vi "parse and execute command.vi"(8 "Python Command":string) -> (1 "Python Return String":string, 2 "exit":bool)   [LabVIEW 2014]
panel:
  in  "base path":path=path "D:/Scripts/VIs/SLLServer/NanonisCommand"
  out "error out":errorcluster
  in  "VI Refnum":refnum<vi>
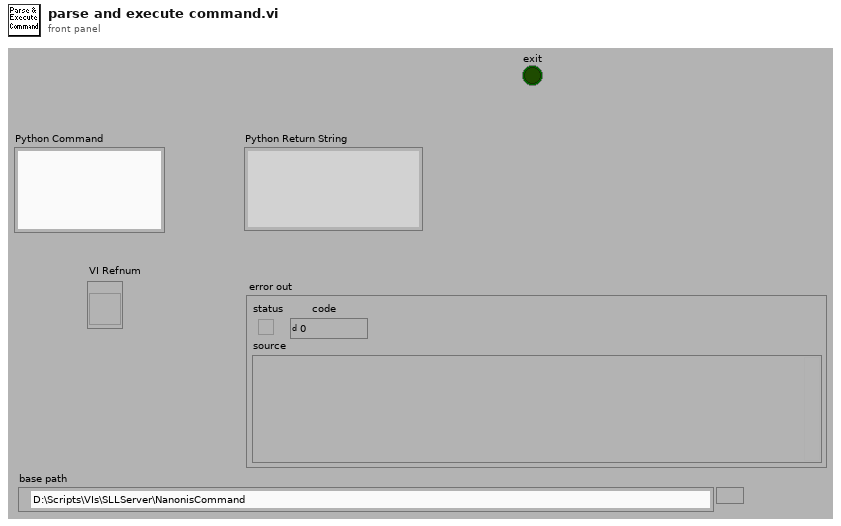
[diagram p1: front panel]
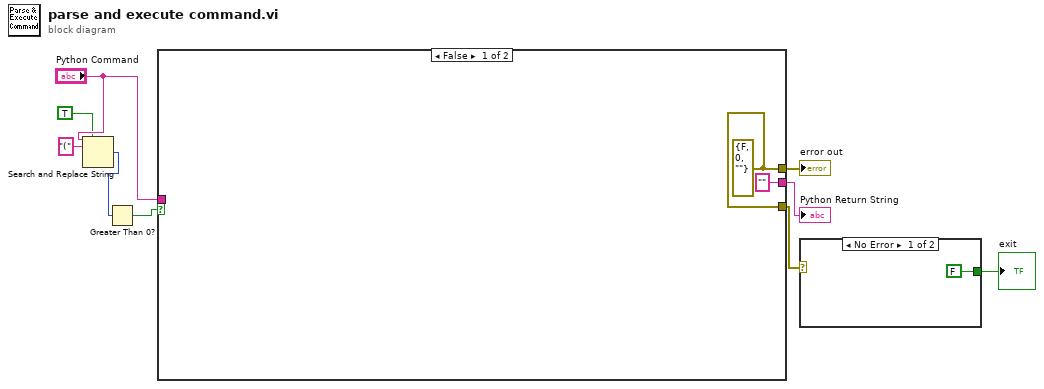
[diagram p0: block diagram]
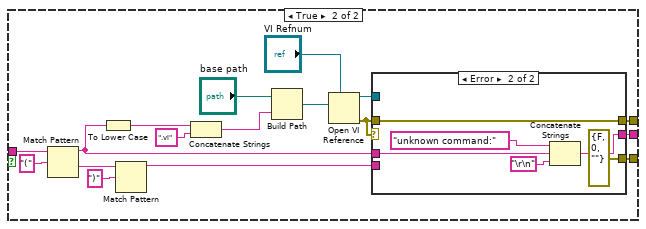
[diagram p2: hidden frame]
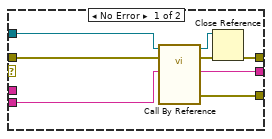
[diagram p3: hidden frame]
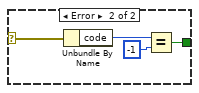
[diagram p4: hidden frame]
diagram:
  n1 = Search and Replace String(replace all?=TRUE ("replace all? (F)"), input string="Python Command", search string="(") -> (number of replacements=w1:i32)  [unwired: 5 in, 3 out]
  n2 = Greater Than 0?(x=w1) -> (x > 0?=w2:bool)
  n3 = case shown="False" w2 {
    tunnel: "Python Command" -> [_ w28]
    tunnel: ["" ("Output") w21] -> w9
    tunnel: [w10 w13] -> w7
    tunnel: [w10 w12] -> w6
    frame False {
      w10 = errorcluster {"status"=FALSE, "code"=0, "source"=""} ("error out")
    }
    frame True {
      n4 = Match Pattern(string=w28, regular expression="(") -> (before substring=w18:string, after substring=w25:string)  [unwired: 1 in, 2 out]
      n5 = To Lower Case(string=w18) -> (all lower case string=w14:string)
      n6 = Match Pattern(string=w25, regular expression=")") -> (before substring=w22:string)  [unwired: 1 in, 3 out]
      n7 = Concatenate Strings(w14, ".vi" ("regular expression")) -> (w16:string)
      n8 = Build Path(base path="base path", name or relative path=w16) -> (appended path=w17:path)
      n9 = Open VI Reference(type specifier VI Refnum (for type only)="VI Refnum", vi path=w17) -> (vi reference=w23:refnum<vi>, error out=w19:errorcluster)  [unwired: 4 in]
      n10 = case shown="Error" w19 {
        tunnel: w23 -> [w36 _]
        tunnel: w19 -> [w34 w42]
        tunnel: [w32 w42] -> w13
        tunnel: w22 -> [w31 _]
        tunnel: [w30 w38] -> w21
        tunnel: w18 -> [_ w41]
        tunnel: [w29 errorcluster {"status"=FALSE, "code"=0, "source"=""} ("error out")] -> w12
        frame No Error {
          n11 = call-by-ref "?"(reference=w36, error in=w34, "Input"=w31) -> (reference out=w35:refnum<vi>, error out=w33:errorcluster, 0:"error out"=w29:errorcluster, "Output"=w30:string)  [unwired: 9 in]
          n12 = Close Reference(reference=w35, error in (no error)=w33) -> (error out=w32:errorcluster)
        }
        frame Error {
          n13 = Concatenate Strings("unknown command:" ("Output"), w41, "\r\n") -> (w38:string)
        }
      }
    }
  }
  "Python Return String" <- w9
  "error out" <- w7
  n14 = case shown="No Error" w6 {
    selector: w6 -> [_ w47]
    tunnel: [FALSE w44] -> w8
    frame No Error {
    }
    frame Error {
      n15 = Unbundle By Name(w47) -> ("code"=w46:i32)
      n16 = Equal?(x=w46, y=-1) -> (x = y?=w44:bool)
    }
  }
  "exit" <- w8
